vi "Cat Head.vi"(8 "error in (no error)":errorcluster, 10 "Numeric":u16, 11 "Ring in":refnum<vi>) -> (0 "error out":errorcluster)   [LabVIEW 2010]
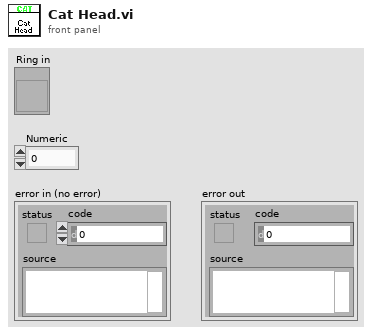
[diagram p1: front panel]
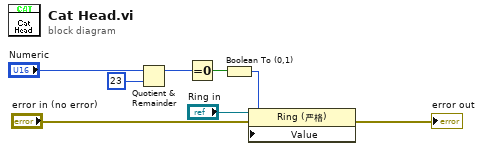
[diagram p0: block diagram]
diagram:
  n1 = Quotient & Remainder(x="Numeric", y=u16 23) -> (x-y*floor(x/y)=w6:u16)  [unwired: 1 out]
  n2 = Equal To 0?(x=w6) -> (x = 0?=w7:bool)
  n3 = Boolean To (0,1)(Boolean=w7) -> (0, 1=w8:i16)
  n4 = property on="Property Node" class="Ring (严格)"(reference="Ring in", error in="error in (no error)", "Value"=w8) -> (error out=→"error out":errorcluster)  [unwired: 1 out]
